vi "SD-File Exists__ogtk.vi"   [LabVIEW 2020, in "SD-openg_file.lvlib"]
doc: "Checks to see whether a path exists on disk and whether it is a directory."
uses:
  SD-openg_file.lvlib
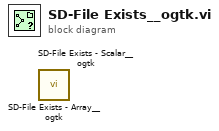
[diagram p0: block diagram]
diagram:
  n1 = call "SD-File Exists - Array__ogtk.vi"() -> ()  [unwired: 7 in, 2 out]
  n2 = call "SD-File Exists - Scalar__ogtk.vi"() -> ()  [unwired: 7 in, 2 out]
